vi "Send Stop.vi"(8 "error in":errorcluster, 10 "Stop":bool, 11 "MCRs":refnum<class "Master CR.lvclass">[](array[class])) -> (0 "error out":errorcluster, 3 "MCRs out":refnum<class "Master CR.lvclass">[](array[class]))   [LabVIEW 2021, in "Master CR.lvclass"]
uses:
  Master CR.lvclass
  Master CR.lvclass/Master CR.ctl
  <vilib>/Utility/error.llb/Clear Errors.vi
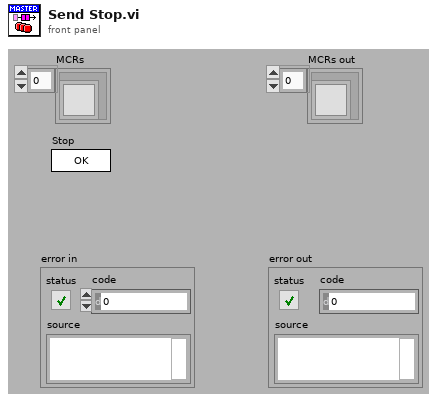
[diagram p1: front panel]
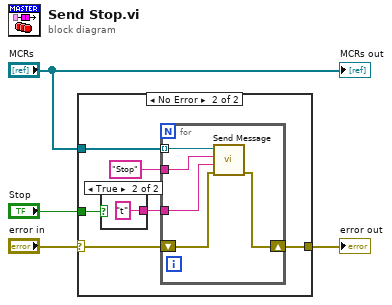
[diagram p0: block diagram]
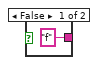
[diagram p3: hidden frame]
diagram:
  n1 = case shown="No Error" "error in" {
    selector: "error in" -> [w5 w11]
    tunnel: [w5 w8] -> w4
    tunnel: "MCRs" -> [_ w6]
    tunnel: "Stop" -> [_ w7]
    frame Error {
    }
    frame No Error {
      n2 = case shown="True" w7 {
        tunnel: ["f" ("Message") "t" ("Message")] -> w9
        frame False {
        }
        frame True {
        }
      }
      n3 = for {
        tunnel: "Stop" ("Message") -> [w18]
        tunnel: w9 -> [w17]
        shift-right: [w16] -> w8
        shift-left: w11 -> [w15]
        tunnel: w6 -> [w14] mode=indexing
        n4 = call "Send Message.vi"("error in (no error)"=w15, "Message Data"=w17, "Message"=w18, "Master CR in"=w14) -> ("error out"=w16:errorcluster)  [unwired: 5 in, 2 out]
      }
    }
  }
  "error out" <- w4
  "MCRs out" <- "MCRs"
